vi "运维调试_氨氮.vi"() -> ()   [LabVIEW 2016, in "斯坦道氨氮.lvlib"]
uses:
  <vilib>/Utility/miscctls.llb/LVPointTypeDef.ctl
  <vilib>/Utility/config.llb/NI_LVConfig.lvlib
  <vilib>/ptbypt/NI_PtbyPt.lvlib
panel:
  in  "仪器参数设置":bool
  in  "模块启用":bool
  in  "串口设置":bool
  in  "备用系数一键写入":bool
  in  "公式一键写入":bool
  in  "流程路径":path=path "C:/Users/STD/Documents/斯坦道流程文件/流程.xml"
  in  "曲线模型":cluster{"X^2":dbl, "X":dbl, "B":dbl}(xcontrol)
  out "字符串":string
  in  "质控参数设置":bool
  in  "自动测试量程配置":T1
  out "温度2":sgl
  out "温度1":sgl
  out "ADC":sgl
  out "固件版本号":string
  in  "数组":string[](array[string])
  in  "备用系数写入":bool
  in  "备用系数读取":bool
  in  "备用系数":T2
  in  "量程切换阈值写入":bool
  in  "量程切换阈值读取":bool
  in  "量程切换阈值":cluster{"阈值":dbl, "标液浓度":dbl}
  in  "参数下拉列表":enum16{"总磷", "总氮", "氨氮"}(ring)=enum."氨氮"
  in  "量程下拉列表":enum16{"低量程", "高量程"}(ring)
  in  "测量模式下拉列表":enum16{"水样测量", "零点核查", "跨度核查", "标样核查", "加标回收"}(ring)
  in  "公式":cluster{"X^2":dbl, "X":dbl, "b":dbl}
  in  "写公式":bool
  in  "读公式":bool
  in  "返回":bool
  in  "设置":bool
  out "序列号":string="序列号"
  out "测量数据":T3(xcontrol)
  out "集成报警信息":string
  out "定时启动":bool
  out "运行状态":T4(xcontrol)
  in  "停止":bool
  in  "手动启动":bool
  in  "单步测试":bool
  in  "总磷氨氮调试":u16[](xcontrol)
  out "F3":sgl format="%#.6f"
  out "F2":sgl format="%#.6f"
  out "F1":sgl format="%#.6f"
  out "F0":sgl format="%#.6f"
  out "多列列表框":i32(listbox)
  # "参数设置"
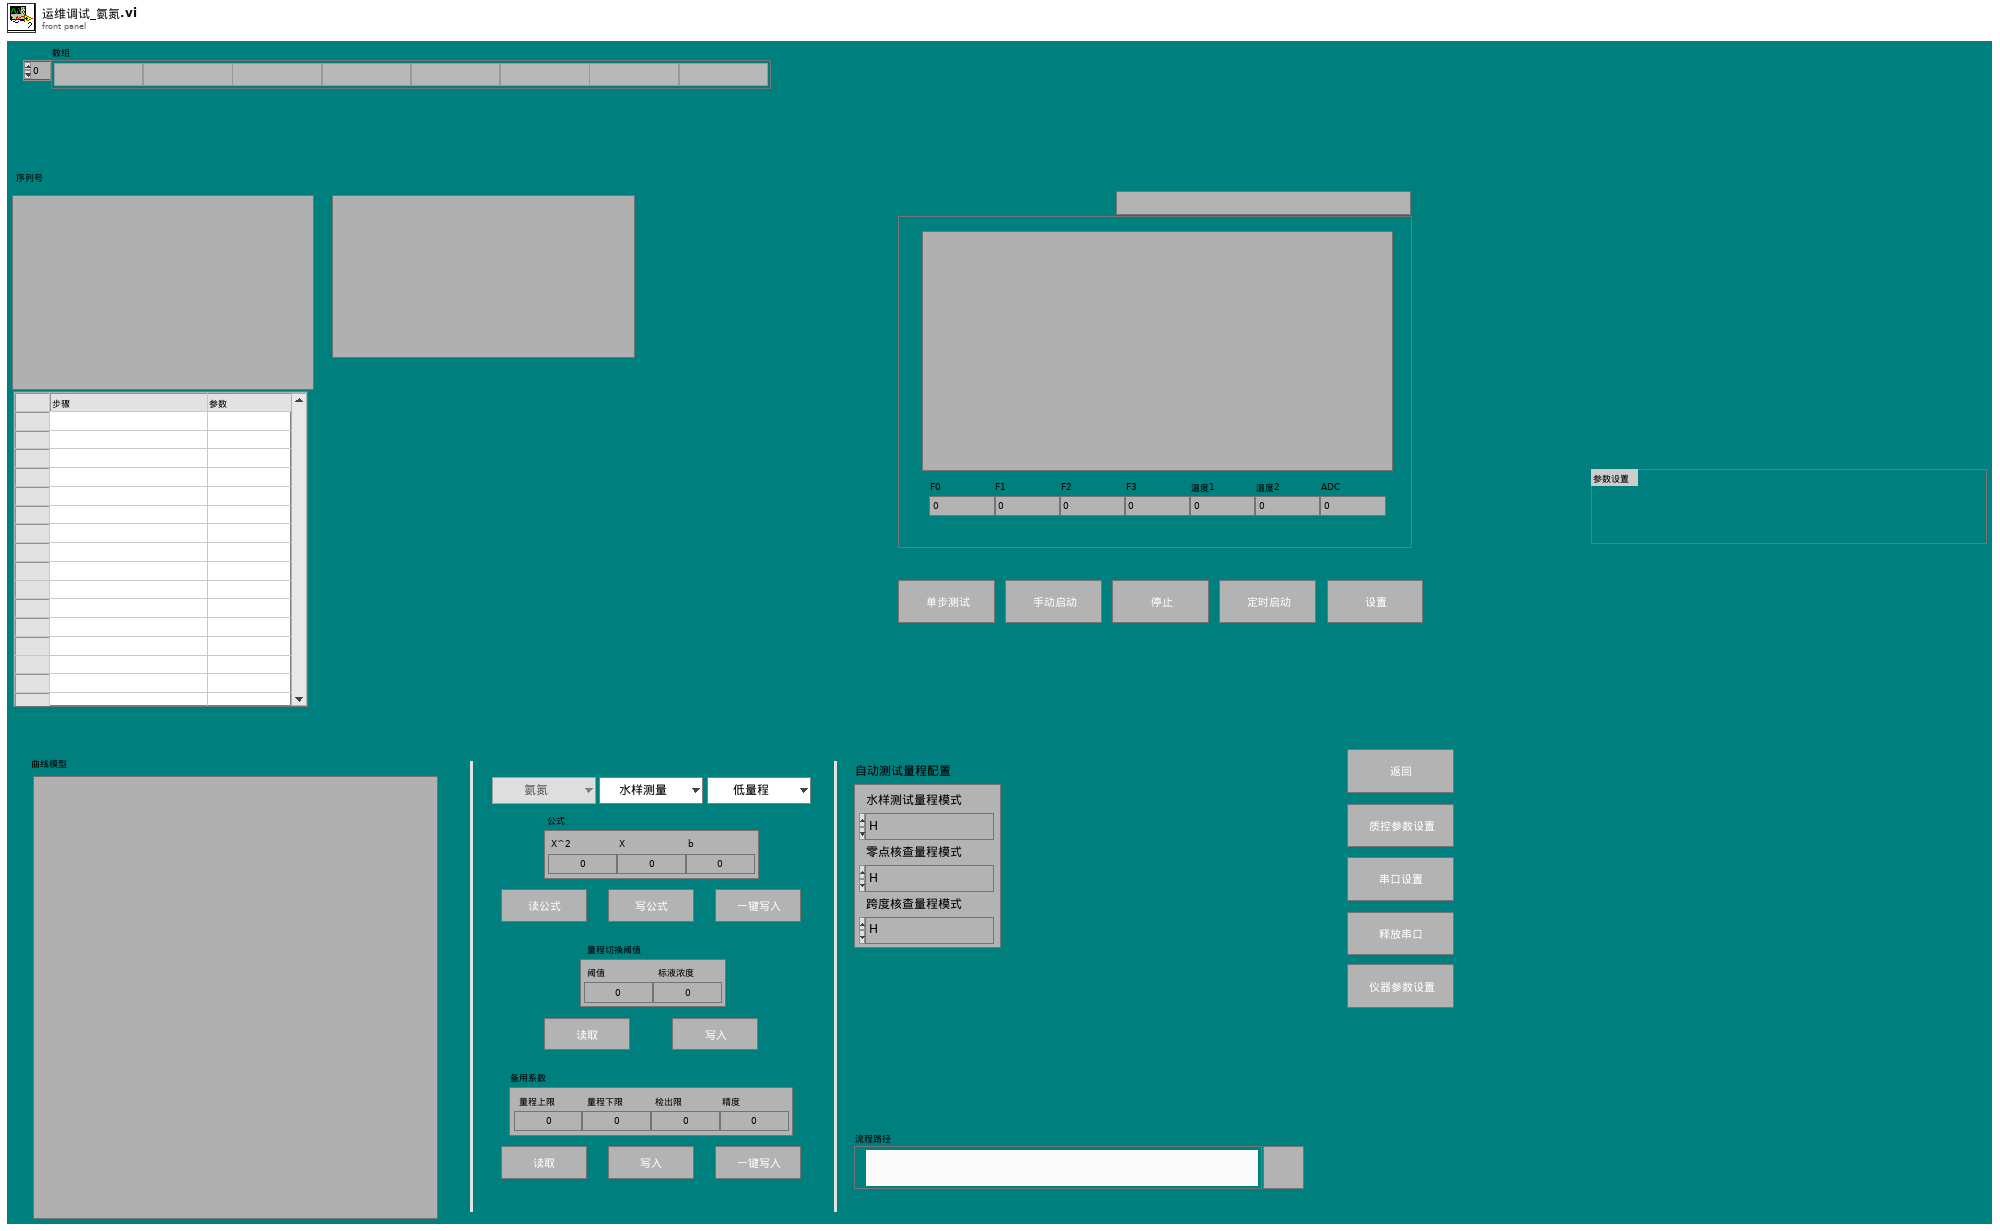
[diagram p1: front panel]
types:
  T1 = cluster{"水样测试量程模式":enum16{"H", "L", "AUTO"}, "空白核查量程模式":enum16{"H", "L", "AUTO"}, "跨度核查量程模式":enum16{"H", "L", "AUTO"}}
  T2 = cluster{"量程上限":dbl, "量程下限":dbl, "检出限":dbl, "精度":dbl}
  T3 = cluster{"flowid":u16, "测量精度":u16, "测量数据区":cluster{"因子编码":u32, "单位":u16, "标样参考值":sgl, "水样数据时间":timestamp, "水样实测值":sgl, "水样数据标识":string, "标样数据时间":timestamp, "标样实测值":sgl, "标样数据标识":string, "空白数据时间":timestamp, "空白实测值":sgl, "空白数据标识":string, "零点核查数据时间":timestamp, "零点核查实测值":sgl, "零点核查数据标识":string, "跨度核查数据时间":timestamp, "跨度核查实测值":sgl, "跨度核查数据标识":string, "加标回收数据时间":timestamp, "加标回收实测值":sgl, "加标回收数据标识":string, "平行样数据时间":timestamp, "平行样实测值":sgl, "平行样数据标识":string, "F0":sgl, "F1":sgl, "F2":sgl, "F3":sgl, "F4":sgl, "F5":sgl, "F6":sgl, "F7":sgl, "温度":sgl, "湿度":sgl, "X值":sgl}}
  T4 = cluster{"系统时间":timestamp, "工作状态":enum16{"空闲", "水样测试", "标样核查", "零点核查", "跨度核查", "空白测试", "平行样测试", "加标回收", "空白校准", "标样校准", "初始化（清洗）"}, "测量模式":enum16{"待机", "连续模式", "周期模式", "定点模式", "受控模式", "手动模式"}, "告警代码":u16, "故障代码":u16, "日志代码":u16, "软件版本":u16, "F0":sgl, "F1":sgl, "F2":sgl, "F3":sgl, "T":sgl, "H":sgl, "id":u16, "flowid":u16, "量程":u16, "总磷控温温度1":sgl, "营养盐控温温度2":sgl, "ADC":sgl}
  T5 = enum16{"启动测量", "标样核查", "零点核查", "跨度核查", "空白测试", "平行样测试", "加标回收", "空白校准", "标样校准", "初始化（清洗）", "停止测试", "仪器重启", "校时", "模式设置", "测量间隔设置"}
  T6 = cluster{"控制命令":enum16{"启动测量", "标样核查", "零点核查", "跨度核查", "空白测试", "平行样测试", "加标回收", "空白校准", "标样校准", "初始化（清洗）", "停止测试", "仪器重启", "校时", "模式设置", "测量间隔设置"}, "周期设置类型":enum16{"定点启动", "间隔启动"}, "定时功能启用":bool, "定时间隔":dbl, "24H周期设置":bool[], "零点核查时间":u16, "跨度核查时间":u16, "质控频次":enum16{"关闭", "每天", "星期一", "星期二", "星期三", "星期四", "星期五", "星期六", "星期日"}}
  T7 = enum16{"关闭", "每天", "星期一", "星期二", "星期三", "星期四", "星期五", "星期六", "星期日"}
  T8 = typedef "LVDateTimeRec.ctl" = cluster{"秒数的小数部分":dbl, "秒":i32, "分":i32, "时":i32, "日":i32, "月":i32, "年":i32, "天数（周）":i32, "天数（年）":i32, "DST":i32}
  T9 = enum16{"空闲", "水样测试", "标样核查", "零点核查", "跨度核查", "空白测试", "平行样测试", "加标回收", "空白校准", "标样校准", "初始化（清洗）"}
  T10 = enum32{"Bad", "Idle", "Run top level", "Running"}
  T11 = typedef "LVPointTypeDef.ctl" = cluster{"Horizontal":i16, "Vertical":i16}
  T12 = cluster{"因子编码":u32, "单位":u16, "标样参考值":sgl, "水样数据时间":timestamp, "水样实测值":sgl, "水样数据标识":string, "标样数据时间":timestamp, "标样实测值":sgl, "标样数据标识":string, "空白数据时间":timestamp, "空白实测值":sgl, "空白数据标识":string, "零点核查数据时间":timestamp, "零点核查实测值":sgl, "零点核查数据标识":string, "跨度核查数据时间":timestamp, "跨度核查实测值":sgl, "跨度核查数据标识":string, "加标回收数据时间":timestamp, "加标回收实测值":sgl, "加标回收数据标识":string, "平行样数据时间":timestamp, "平行样实测值":sgl, "平行样数据标识":string, "F0":sgl, "F1":sgl, "F2":sgl, "F3":sgl, "F4":sgl, "F5":sgl, "F6":sgl, "F7":sgl, "温度":sgl, "湿度":sgl, "X值":sgl}
  T13 = typedef "NI_LVConfig.lvlib/Config Data RefNum.ctl" = refnum<k1>
  T14 = cluster{"参数下拉列表":enum16{"总磷", "总氮", "氨氮"}, "测量模式下拉列表":enum16{"水样测量", "零点核查", "跨度核查", "标样核查", "加标回收"}, "量程下拉列表":enum16{"低量程", "高量程"}}
  T15 = cluster{"启动模式":enum16{"跨度核查", "水样测量", "空白核查", "标样核查", "加标回收"}, "启动参数":u16, "量程":enum16{"低量程", "高量程"}}
  T16 = cluster{"时间标识":timestamp, "设备":string, "日志信息":string, "流程参数":string}
  T17 = cluster{"时间标识":timestamp, "设备":string, "日志信息":string}
  T18 = typedef "LVRowAndColumnUnsignedTypeDef.ctl" = cluster{"Row":u32, "Column":u32}
  T19 = cluster{"站号":u16, "量程切换":enum32{"H", "L", "AUTO"}, "控制命令":enum16{"启动测量", "标样核查", "零点核查", "跨度核查", "空白测试", "平行样测试", "加标回收", "空白校准", "标样校准", "初始化（清洗）", "停止测试", "仪器重启", "校时", "模式设置", "测量间隔设置"}, "模式设置":enum16{"待机", "连续模式", "周期模式", "定点模式", "受控模式", "手动模式"}, "测量间隔":u16}
  T20 = cluster{"氨氮跨度值":dbl, "氨氮零点标准液浓度":dbl, "氨氮跨度标准液浓度":dbl, "氨氮标准液标准浓度":dbl}
  T21 = cluster{"确定":bool, "跨度值":dbl, "零点标准液浓度":dbl, "跨度标准液浓度":dbl, "标准液标准浓度":dbl}
  T22 = cluster{"测量量程":dbl, "测量精度":dbl, "测量间隔":dbl, "消解温度":dbl, "消解时长":dbl, "空白校准时间":timestamp, "曲线截距":dbl, "曲线斜率":dbl, "测量检出限":dbl, "测量信号值":dbl, "线性相关系数":dbl, "二次多项式系数":dbl, "标样校准时间":timestamp, "单位":u16}
  T23 = cluster{"确定":bool, "测量量程":dbl, "测量精度":dbl, "测量间隔":dbl, "消解温度":dbl, "消解时长":dbl, "空白校准时间":timestamp, "曲线截距":dbl, "曲线斜率":dbl, "测量检出限":dbl, "测量信号值":dbl, "线性相关系数":dbl, "二次多项式系数":dbl, "标样校准时间":timestamp, "单位":u16}
  T24 = cluster{"控制命令":enum16{"启动测量", "标样核查", "零点核查", "跨度核查", "空白测试", "平行样测试", "加标回收", "空白校准", "标样校准", "初始化（清洗）", "停止测试", "仪器重启", "校时", "模式设置", "测量间隔设置"}, "周期设置类型":enum16{"定点启动", "间隔启动"}, "定时功能启用":bool, "定时间隔":dbl, "24H周期设置":bool[], "空白核查时间":u16, "跨度核查时间":u16, "质控频次":enum16{"关闭", "每天", "星期一", "星期二", "星期三", "星期四", "星期五", "星期六", "星期日"}}
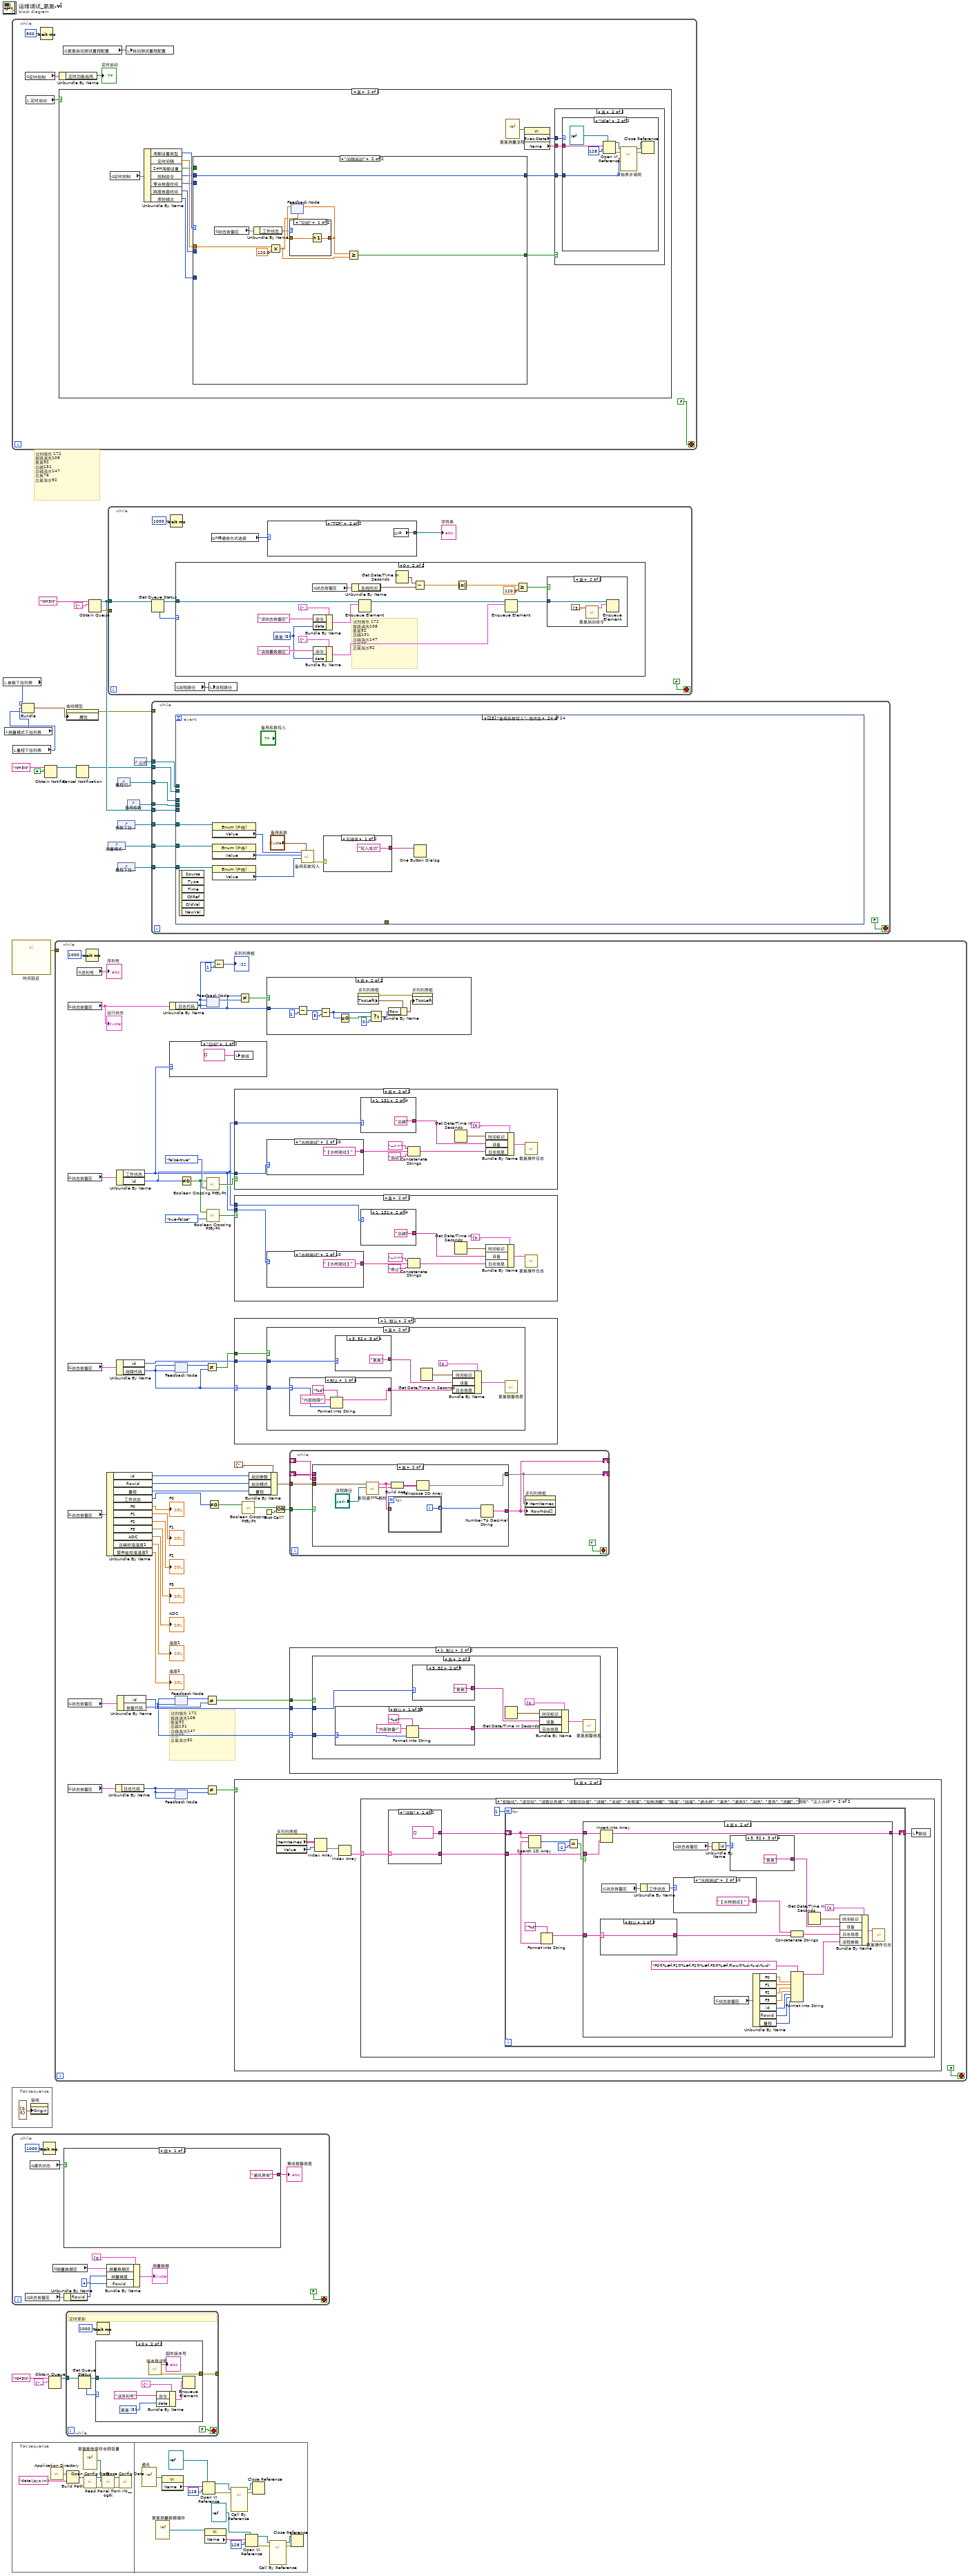
[diagram p0: block diagram]
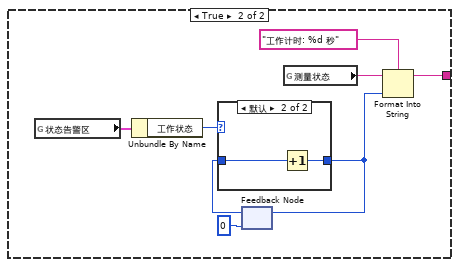
[diagram p3: hidden frame]
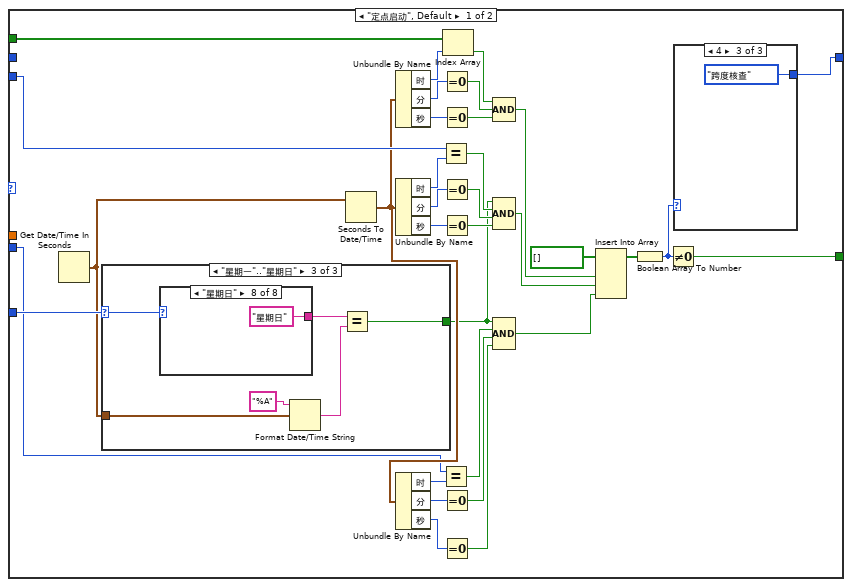
[diagram p8: hidden frame]
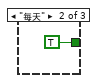
[diagram p10: hidden frame]
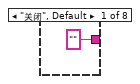
[diagram p11: hidden frame]
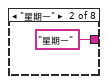
[diagram p12: hidden frame]
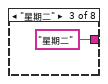
[diagram p13: hidden frame]
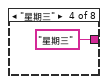
[diagram p14: hidden frame]
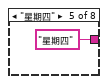
[diagram p15: hidden frame]
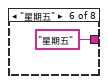
[diagram p16: hidden frame]
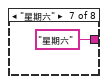
[diagram p17: hidden frame]
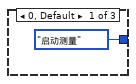
[diagram p18: hidden frame]
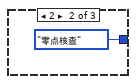
[diagram p19: hidden frame]
diagram:
  # "试剂填充 172 \n管路清洗108\n氨氮92\n总磷131\n总磷海水147\n总氮76\n总氮海水92"
  n1 = local read "参数下拉列表"() -> (w4:enum16{"总磷", "总氮", "氨氮"})
  n2 = local read "测量模式下拉列表"() -> (w3:enum16{"水样测量", "零点核查", "跨度核查", "标样核查", "加标回收"})
  n3 = while {
    stop <- FALSE stop-if-true
    n4 = global read "氨氮断电保存全局变量.vi" "定时控制"() -> (w25:T6)
    n5 = local read "定时启动"() -> (w27:bool)
    n6 = Wait (ms)(milliseconds to wait=u32 500 ("等待时间（毫秒）")) -> ()  [unwired: 1 out]
    n7 = Unbundle By Name(w25) -> ("定时功能启用"=→"定时启动":bool)
    n8 = case shown="真" w27 {
      frame False {
      }
      frame True {
        n9 = global read "氨氮断电保存全局变量.vi" "定时控制"() -> (w42:T6)
        n10 = Unbundle By Name(w42) -> ("周期设置类型"=w41:enum16{"定点启动", "间隔启动"}, "定时间隔"=w40:dbl, "24H周期设置"=w39:bool[], "控制命令"=w34:T5, "零点核查时间"=w32:u16, "跨度核查时间"=w31:u16, "质控频次"=w30:T7)
        n11 = case shown="\"间隔启动\"" w41 {
          tunnel: w40 -> [_ w111]
          tunnel: w39 -> [w77 _]
          tunnel: [w55 w109] -> w38
          tunnel: w34 -> [_ w107]
          tunnel: [w81 w107] -> w33
          tunnel: w30 -> [w80 _]
          tunnel: w32 -> [w73 _]
          tunnel: w31 -> [w62 _]
          frame "定点启动", Default {
            n12 = Get Date/Time In Seconds() -> (seconds since 1Jan1904=w79:timestamp)
            n13 = case shown="\"星期一\"..\"星期日\"" w80 {
              selector: w80 -> [_ _ w91]
              tunnel: w79 -> [_ _ w92]
              tunnel: [_ TRUE w88] -> w61
              frame "关闭", Default {
              }
              frame "每天" {
              }
              frame "星期一".."星期日" {
                n14 = case shown="\"星期日\"" w91 {
                  tunnel: ["" ("时间格式字符串(%c)") "星期一" ("时间格式字符串(%c)") "星期二" ("时间格式字符串(%c)") "星期三" ("时间格式字符串(%c)") "星期四" ("时间格式字符串(%c)") "星期五" ("时间格式字符串(%c)") "星期六" ("时间格式字符串(%c)") "星期日" ("时间格式字符串(%c)")] -> w90
                  frame "关闭", Default {
                  }
                  frame "星期一" {
                  }
                  frame "星期二" {
                  }
                  frame "星期三" {
                  }
                  frame "星期四" {
                  }
                  frame "星期五" {
                  }
                  frame "星期六" {
                  }
                  frame "星期日" {
                  }
                }
                n15 = Format Date/Time String(time format string (%c)="%A" ("时间格式字符串(%c)"), seconds (now)=w92) -> (date/time string=w89:string)  [unwired: 1 in]
                n16 = Equal?(x=w90, y=w89) -> (x = y?=w88:bool)
              }
            }
            n17 = Seconds To Date/Time(time stamp (now)=w79) -> (date time rec=w63:T8)  [unwired: 1 in]
            n18 = Unbundle By Name(w63) -> ("时"=w86:i32, "分"=w84:i32, "秒"=w85:i32)
            n19 = Unbundle By Name(w63) -> ("时"=w74:i32, "分"=w76:i32, "秒"=w75:i32)
            n20 = Unbundle By Name(w63) -> ("时"=w66:i32, "分"=w64:i32, "秒"=w65:i32)
            n21 = Equal?(x=w73, y=w74) -> (x = y?=w72:bool)
            n22 = Equal?(x=w62, y=w66) -> (x = y?=w67:bool)
            n23 = Equal To 0?(x=w84) -> (x = 0?=w83:bool)
            n24 = Equal To 0?(x=w85) -> (x = 0?=w82:bool)
            n25 = Equal To 0?(x=w76) -> (x = 0?=w71:bool)
            n26 = Equal To 0?(x=w75) -> (x = 0?=w70:bool)
            n27 = Equal To 0?(x=w64) -> (x = 0?=w68:bool)
            n28 = Equal To 0?(x=w65) -> (x = 0?=w69:bool)
            n29 = Index Array(array=w77, index=w86) -> (element=w78:bool)
            n30 = Compound Arithmetic op=AND ("复合运算")(w78, w83, w82) -> (w59:bool)
            n31 = Compound Arithmetic op=AND ("复合运算")(w61, w72, w71, w70) -> (w58:bool)
            n32 = Compound Arithmetic op=AND ("复合运算")(w61, w67, w68, w69) -> (w57:bool)
            n33 = Insert Into Array(array=bool[] [], new element #1=w59, new element #2=w58, new element #3=w57) -> (w56:bool[])  [unwired: 1 in]
            n34 = Boolean Array To Number(Boolean array=w56) -> (number=w54:u32)
            n35 = Not Equal To 0?(x=w54) -> (x != 0?=w55:bool)
            n36 = case shown="4" w54 {
              tunnel: [T5."启动测量" ("控制命令") T5."零点核查" ("控制命令") T5."跨度核查" ("控制命令")] -> w81
              frame 0, Default {
              }
              frame 2 {
              }
              frame 4 {
              }
            }
          }
          frame "间隔启动" {
            n37 = global read "VAR氨氮全局变量.vi" "状态告警区"() -> (w106:T4)
            n38 = Unbundle By Name(w106) -> ("工作状态"=w105:T9)
            n39 = Multiply(x=w111, y=120.0) -> (x*y=w108:dbl)
            n40 = feedback #1(w108) -> (w113:dbl)
            n41 = case shown="\"空闲\"" w105 {
              tunnel: w113 -> [w115 _]
              tunnel: [w114 _] -> w112
              frame "空闲" {
                n42 = Increment(x=w115) -> (x+1=w114:dbl)
              }
              frame "水样测试", Default {
              }
            }
            n43 = feedback-in #1(w112) -> ()
            n44 = Greater Or Equal?(x=w112, y=w108) -> (x >= y?=w109:bool)
          }
        }
        n45 = vi-ref "氨氮测量流程.vi"() -> (w37:refnum<vi>)
        n46 = property class="VI"(reference=w37) -> ("Exec.State"=w36:T10, "Name"=w35:string)  [unwired: 1 in, 2 out]
        n47 = case shown="真" w38 {
          tunnel: w35 -> [_ w45]
          tunnel: w33 -> [_ w44]
          tunnel: w36 -> [_ w43]
          frame False {
          }
          frame True {
            n48 = case shown="\"Idle\"" w43 {
              tunnel: w45 -> [_ w49]
              tunnel: w44 -> [_ w47]
              frame "Bad", Default {
              }
              frame "Idle" {
                n49 = Open VI Reference(type specifier VI Refnum (for type only)=refnum<vi> refnum, vi path=w49, options=128 ("选项")) -> (vi reference=w50:refnum<vi>, error out=w51:errorcluster)  [unwired: 3 in]
                n50 = call-by-ref "开始异步调用"(reference=w50, error in=w51, "控制命令"=w47) -> (reference out=w52:refnum<vi>, error out=w53:errorcluster)  [unwired: 11 in]
                n51 = Close Reference(reference=w52, error in (no error)=w53) -> ()  [unwired: 1 out]
              }
            }
          }
        }
      }
    }
    n52 = global read "氨氮断电保存全局变量.vi" "氨氮自动测试量程配置"() -> (w26:T1)
    n53 = local write "自动测试量程配置"(w26) -> ()
  }
  n54 = call "时间延迟"() -> ("error out"=w13:errorcluster)  [unwired: 11 in]
  n55 = flat-sequence {
    frame #0 {
      n56 = property on="窗格" class="Pane"("Origin"=T11 {"Horizontal"=0, "Vertical"=0} ("原点")) -> ()  [unwired: 2 in, 2 out]
    }
  }
  n57 = while {
    stop <- FALSE stop-if-true
    n58 = global read "VAR氨氮全局变量.vi" "状态告警区"() -> (w122:T4)
    n59 = global read "VAR氨氮全局变量.vi" "通讯状态"() -> (w124:bool)
    n60 = Wait (ms)(milliseconds to wait=u32 1000 ("等待时间（毫秒）")) -> ()  [unwired: 1 out]
    n61 = global read "VAR氨氮全局变量.vi" "测量数据区"() -> (w117:T12)
    n62 = case shown="假" w124 {
      tunnel: ["通讯异常" ("集成报警信息") w129] -> w123
      frame False {
      }
      frame True {
        n63 = global read "VAR氨氮全局变量.vi" "状态告警区"() -> (w135:T4)
        n64 = Unbundle By Name(w135) -> ("工作状态"=w134:T9)
        n65 = feedback #2(0) -> (w132:i32)
        n66 = case shown="默认" w134 {
          tunnel: w132 -> [_ w137]
          tunnel: [_ w136] -> w130
          frame "空闲" {
          }
          frame Default {
            n67 = Increment(x=w137) -> (x+1=w136:i32)
          }
        }
        n68 = feedback-in #2(w130) -> ()
        n69 = global read "VAR氨氮全局变量.vi" "测量状态"() -> (w128:string)
        n70 = Format Into String(format string="工作计时: %d 秒" ("格式字符串"), initial string=w128, w130) -> (resulting string=w129:string)  [unwired: 1 in, 1 out]
      }
    }
    "集成报警信息" <- w123
    n71 = Unbundle By Name(w122) -> ("flowid"=w121:u16)
    n72 = Bundle By Name(cluster=T3 {"flowid"=0, "测量精度"=0, "测量数据区"={"因子编码"=0, "单位"=0, "标样参考值"=0.0, "水样数据时间"=timestamp(0 s since 1904-01-01), "水样实测值"=0.0, "水样数据标识"="", "标样数据时间"=timestamp(0 s since 1904-01-01), "标样实测值"=0.0, "标样数据标识"="", "空白数据时间"=timestamp(0 s since 1904-01-01), "空白实测值"=0.0, "空白数据标识"="", "零点核查数据时间"=timestamp(0 s since 1904-01-01), "零点核查实测值"=0.0, "零点核查数据标识"="", "跨度核查数据时间"=timestamp(0 s since 1904-01-01), "跨度核查实测值"=0.0, "跨度核查数据标识"="", "加标回收数据时间"=timestamp(0 s since 1904-01-01), "加标回收实测值"=0.0, "加标回收数据标识"="", "平行样数据时间"=timestamp(0 s since 1904-01-01), "平行样实测值"=0.0, "平行样数据标识"="", "F0"=0.0, "F1"=0.0, "F2"=0.0, "F3"=0.0, "F4"=0.0, "F5"=0.0, "F6"=0.0, "F7"=0.0, "温度"=0.0, "湿度"=0.0, "X值"=0.0}} ("总氮测量数据"), "测量数据区"=w117, "测量精度"=u16 4, "flowid"=w121) -> (→"测量数据":T3)
  }
  n73 = flat-sequence {
    frame #0 {
      n74 = call <vilib>:"Application Directory.vi"() -> ("Application Directory"=w145:path)
      n75 = Build Path(base path=w145, name or relative path="data\\sys.ini" ("名称或相对路径")) -> (appended path=w143:path)
      n76 = vi-ref "氨氮断电保存全局变量.vi"() -> (w141:refnum<vi>)
      n77 = call <vilib>:"Open Config Data.vi"("configuration file path"=w143) -> ("error out"=w139:errorcluster, "refnum"=w142:T13)  [unwired: 8 in, 1 out]
      n78 = call <userlib>:"Read Panel from INI__ogtk.vi"("error in (no error)"=w139, "VI ref"=w141, "refnum"=w142) -> ("error out"=w138:errorcluster, "refnum out"=w140:T13)  [unwired: 7 in]
      n79 = call <vilib>:"Close Config Data.vi"("error in (no error)"=w138, "refnum"=w140) -> ()  [unwired: 8 in, 2 out]
    }
    frame #1 {
      n80 = vi-ref "通讯.vi"() -> (w161:refnum<vi>)
      n81 = vi-ref "氨氮测量数据储存.vi"() -> (w153:refnum<vi>)
      n82 = property class="VI"(reference=w161) -> ("Name"=w160:string)  [unwired: 1 in, 2 out]
      n83 = Open VI Reference(type specifier VI Refnum (for type only)=refnum<vi> refnum, vi path=w160, options=128 ("选项")) -> (vi reference=w158:refnum<vi>, error out=w156:errorcluster)  [unwired: 3 in]
      n84 = property class="VI"(reference=w153) -> ("Name"=w146:string)  [unwired: 1 in, 2 out]
      n85 = call-by-ref "?"(reference=w158, error in=w156) -> (reference out=w154:refnum<vi>, error out=w155:errorcluster)  [unwired: 12 in]
      n86 = Open VI Reference(type specifier VI Refnum (for type only)=refnum<vi> refnum, vi path=w146, options=128 ("选项")) -> (vi reference=w148:refnum<vi>, error out=w150:errorcluster)  [unwired: 3 in]
      n87 = Close Reference(reference=w154, error in (no error)=w155) -> ()  [unwired: 1 out]
      n88 = call-by-ref "?"(reference=w148, error in=w150) -> (reference out=w152:refnum<vi>, error out=w151:errorcluster)  [unwired: 12 in]
      n89 = Close Reference(reference=w152, error in (no error)=w151) -> ()  [unwired: 1 out]
    }
  }
  n90 = local read "量程下拉列表"() -> (w2:enum16{"低量程", "高量程"})
  n91 = Bundle("参数下拉列表"=w4, "测量模式下拉列表"=w3, "量程下拉列表"=w2) -> (w1:T14)  [unwired: 1 in]
  n92 = Obtain Notifier(name (unnamed)="NH3N" ("名称（未命名）"), notification data type=FALSE) -> (notifier out=w6:refnum<notifier>)  [unwired: 2 in, 2 out]
  n93 = Obtain Queue(name (unnamed)="NH3N" ("名称（未命名）"), element data type=cluster{"命令":string, "data":variant} {"命令"="", "data"=variant}) -> (queue out=w10:refnum<queue>)  [unwired: 3 in, 2 out]
  n94 = while {
    tunnel: w13 -> [_]
    stop <- FALSE stop-if-true
    # "试剂填充 172 \n管路清洗108\n氨氮92\n总磷131\n总磷海水147\n总氮76\n总氮海水92"
    n95 = global read "VAR氨氮全局变量.vi" "状态告警区"() -> (w195:T4)
    "运行状态" <- w195
    n96 = global read "VAR氨氮全局变量.vi" "状态告警区"() -> (w182:T4)
    n97 = global read "VAR氨氮全局变量.vi" "状态告警区"() -> (w187:T4)
    n98 = global read "VAR氨氮全局变量.vi" "状态告警区"() -> (w203:T4)
    n99 = global read "VAR氨氮全局变量.vi" "状态告警区"() -> (w192:T4)
    n100 = global read "VAR氨氮全局变量.vi" "状态告警区"() -> (w180:T4)
    n101 = global read "VAR氨氮全局变量.vi" "序列号"() -> (→"序列号":string)
    n102 = Wait (ms)(milliseconds to wait=u32 1000 ("等待时间（毫秒）")) -> ()  [unwired: 1 out]
    n103 = Unbundle By Name(w203) -> ("id"=w200:u16, "flowid"=w202:u16, "量程"=w201:u16, "工作状态"=w170:T9, "F0"=→"F0":sgl, "F1"=→"F1":sgl, "F2"=→"F2":sgl, "F3"=→"F3":sgl, "ADC"=→"ADC":sgl, "总磷控温温度1"=→"温度1":sgl, "营养盐控温温度2"=→"温度2":sgl)
    n104 = Unbundle By Name(w180) -> ("日志代码"=w179:u16)
    n105 = Unbundle By Name(w182) -> ("工作状态"=w166:T9, "id"=w165:u16)
    n106 = Unbundle By Name(w187) -> ("id"=w186:u16, "故障代码"=w183:u16)
    n107 = Unbundle By Name(w192) -> ("id"=w191:u16, "告警代码"=w188:u16)
    n108 = Unbundle By Name(w195) -> ("日志代码"=w176:u16)
    n109 = case shown="\"空闲\"" w166 {
      frame "空闲" {
        n110 = local write "数组"(string[] [] ("数组")) -> ()
      }
      frame "水样测试", Default {
      }
    }
    n111 = feedback #3(w183) -> (w184:u16)
    n112 = feedback-in #3(w183) -> ()
    n113 = feedback #4(w188) -> (w189:u16)
    n114 = feedback-in #4(w188) -> ()
    n115 = feedback #5(w179) -> (w181:u16)
    n116 = feedback-in #5(w179) -> ()
    n117 = Not Equal To 0?(x=w165) -> (x != 0?=w163:bool)
    n118 = Not Equal?(x=w184, y=w183) -> (x != y?=w185:bool)
    n119 = Not Equal?(x=w189, y=w188) -> (x != y?=w190:bool)
    n120 = Not Equal?(x=w179, y=w181) -> (x != y?=w178:bool)
    n121 = feedback-in #6(w176) -> ()
    n122 = feedback #6(w176) -> (w208:u16)
    n123 = call <vilib>:"Boolean Crossing PtByPt.vi"("direction"=enum16{"either", "false-true", "true-false"}."false-true", "input"=w163) -> ("crossing"=w167:bool)  [unwired: 1 in]
    n124 = call <vilib>:"Boolean Crossing PtByPt.vi"("direction"=enum16{"either", "false-true", "true-false"}."true-false", "input"=w163) -> ("crossing"=w162:bool)  [unwired: 1 in]
    n125 = Not Equal To 0?(x=w170) -> (x != 0?=w205:bool)
    n126 = Subtract(x=w176, y=1) -> (x-y=→"多列列表框":i32)
    n127 = case shown="真" w167 {
      tunnel: w165 -> [_ w235]
      tunnel: w166 -> [_ w234]
      frame False {
      }
      frame True {
        n128 = case shown="\"水样测试\"" w234 {
          tunnel: [_ "【水样测试】" ("字符串") "【标样核查】" ("字符串") "【零点核查】" ("字符串") "【跨度核查】" ("字符串") "【空白测试】" ("字符串") "【平行样测试】" ("字符串") "【加标回收】" ("字符串") "【空白校准】" ("字符串") "【标样校准】" ("字符串")] -> w239
          frame "空闲", Default {
          }
          frame "水样测试" {
          }
          frame "标样核查" {
          }
          frame "零点核查" {
          }
          frame "跨度核查" {
          }
          frame "空白测试" {
          }
          frame "平行样测试" {
          }
          frame "加标回收" {
          }
          frame "空白校准" {
          }
          frame "标样校准" {
          }
        }
        n129 = case shown="1, 131" w235 {
          tunnel: [_ "总磷" ("table输入") "氨氮" ("table输入") "总氮" ("table输入")] -> w240
          frame Default {
          }
          frame 1, 131 {
          }
          frame 3, 92 {
          }
          frame 2, 76 {
          }
        }
        n130 = Concatenate Strings("-->>" ("字符串"), w239, "启动" ("字符串")) -> (w238:string)
        n131 = Get Date/Time In Seconds() -> (seconds since 1Jan1904=w241:timestamp)
        n132 = Bundle By Name(cluster=T16 {"时间标识"=timestamp(0 s since 1904-01-01), "设备"="", "日志信息"="", "流程参数"=""} ("data in"), "时间标识"=w241, "设备"=w240, "日志信息"=w238) -> (w233:T16)
        n133 = call "氨氮操作日志.vi"("data in"=w233) -> ()  [unwired: 11 in]
      }
    }
    n134 = case shown="真" w162 {
      tunnel: w165 -> [_ w213]
      tunnel: w166 -> [_ w212]
      frame False {
      }
      frame True {
        n135 = case shown="\"水样测试\"" w212 {
          tunnel: [_ "【水样测试】" ("字符串") "【标样核查】" ("字符串") "【零点核查】" ("字符串") "【跨度核查】" ("字符串") "【空白测试】" ("字符串") "【平行样测试】" ("字符串") "【加标回收】" ("字符串") "【空白校准】" ("字符串") "【标样校准】" ("字符串")] -> w217
          frame "空闲", Default {
          }
          frame "水样测试" {
          }
          frame "标样核查" {
          }
          frame "零点核查" {
          }
          frame "跨度核查" {
          }
          frame "空白测试" {
          }
          frame "平行样测试" {
          }
          frame "加标回收" {
          }
          frame "空白校准" {
          }
          frame "标样校准" {
          }
        }
        n136 = case shown="1, 131" w213 {
          tunnel: [_ "总磷" ("table输入") "氨氮" ("table输入") "总氮" ("table输入")] -> w218
          frame Default {
          }
          frame 1, 131 {
          }
          frame 3, 92 {
          }
          frame 2, 76 {
          }
        }
        n137 = Concatenate Strings("-->>" ("字符串"), w217, "停止" ("字符串")) -> (w216:string)
        n138 = Get Date/Time In Seconds() -> (seconds since 1Jan1904=w219:timestamp)
        n139 = Bundle By Name(cluster=T16 {"时间标识"=timestamp(0 s since 1904-01-01), "设备"="", "日志信息"="", "流程参数"=""} ("data in"), "时间标识"=w219, "设备"=w218, "日志信息"=w216) -> (w211:T16)
        n140 = call "氨氮操作日志.vi"("data in"=w211) -> ()  [unwired: 11 in]
      }
    }
    n141 = case shown="1, 默认" w183 {
      selector: w183 -> [_ w323]
      tunnel: w186 -> [_ w324]
      tunnel: w185 -> [_ w322]
      frame 0 {
      }
      frame 1, Default {
        n142 = case shown="真" w322 {
          tunnel: w324 -> [_ w331]
          tunnel: w323 -> [_ w326]
          frame False {
          }
          frame True {
            n143 = case shown="默认" w326 {
              selector: w326 -> [w333 _ _ _ _ _]
              tunnel: [w332 "无故障" "电机故障" "温度故障" "通讯故障" "滴定故障"] -> w325
              frame Default {
                n144 = Format Into String(format string="%d" ("格式字符串"), initial string="内部故障-" ("工作状态"), w333) -> (resulting string=w332:string)  [unwired: 1 in, 1 out]
              }
              frame 0 {
              }
              frame 1 {
              }
              frame 2 {
              }
              frame 3 {
              }
              frame 4 {
              }
            }
            n145 = case shown="3, 92" w331 {
              tunnel: [_ "总磷" ("table输入") "氨氮" ("table输入") "总氮" ("table输入")] -> w327
              frame Default {
              }
              frame 1, 131 {
              }
              frame 3, 92 {
              }
              frame 2, 76 {
              }
            }
            n146 = Get Date/Time In Seconds() -> (seconds since 1Jan1904=w328:timestamp)
            n147 = Bundle By Name(cluster=T17 {"时间标识"=timestamp(0 s since 1904-01-01), "设备"="", "日志信息"=""} ("data in"), "时间标识"=w328, "设备"=w327, "日志信息"=w325) -> (w329:T17)
            n148 = call "氨氮报警信息.vi"("data in"=w329) -> ()  [unwired: 10 in, 1 out]
          }
        }
      }
    }
    n149 = case shown="真" w178 {
      frame False {
      }
      frame True {
        n150 = property on="多列列表框" class="MCListbox (严格)"() -> ("ItemNames"=w258:string[][], "Value"=w259:i32)  [unwired: 2 in, 2 out]
        n151 = Index Array(array=w258, index (row)=w259) -> (element=w257:string[])  [unwired: 1 in]
        n152 = Index Array(array=w257) -> (element=w256:string)  [unwired: 1 in]
        n153 = case shown="\"初始化\", \"读空白\", \"读取比色值\", \"读取空白值\", \"读数\", \"关阀\", \"关恒温\", \"加热消解\", \"降温\", \"结束\", \"进水样\", \"清洗\", \"清洗1\", \"润洗\", \"显色\", \"消解\", \"预热\", \"注入水样\"" w256 {
          selector: w256 -> [_ w262]
          frame Default {
          }
          frame "初始化", "读空白", "读取比色值", "读取空白值", "读数", "关阀", "关恒温", "加热消解", "降温", "结束", "进水样", "清洗", "清洗1", "润洗", "显色", "消解", "预热", "注入水样" {
            n154 = case shown="\"读数\"" w262 {
              selector: w262 -> [w266 w268]
              tunnel: [w266 w268] -> w261
              tunnel: [string[] [] ("数组") "数组"] -> w260
              frame "读数" {
              }
              frame Default {
              }
            }
            n155 = for {
              N: 1 -> [_]
              tunnel: w261 -> [w270]
              shift-right: [w269] -> w263
              shift-left: w260 -> [w271]
              n156 = Search 1D Array(1D array=w271, element=w270) -> (index of element=w274:i32)  [unwired: 1 in]
              n157 = Format Into String(format string="%s" ("格式字符串"), w270) -> (resulting string=w275:string)  [unwired: 2 in, 1 out]
              n158 = Equal?(x=w274, y=-1) -> (x = y?=w272:bool)
              n159 = case shown="真" w272 {
                tunnel: w275 -> [_ w283]
                tunnel: w271 -> [w277 w287]
                tunnel: w270 -> [_ w286]
                tunnel: [w277 w285] -> w269
                frame False {
                }
                frame True {
                  n160 = Insert Into Array(array=w287, new element=w286) -> (w285:string[])  [unwired: 1 in]
                  n161 = case shown="默认" w283 {
                    selector: w283 -> [w312 w315 w318]
                    tunnel: [w312 w314 w317] -> w282
                    frame Default {
                    }
                    frame "初始化" {
                      n162 = Concatenate Strings("-->>" ("字符串"), w315) -> (w314:string)
                    }
                    frame "结束" {
                      n163 = Concatenate Strings("-->>" ("字符串"), w318) -> (w317:string)
                    }
                  }
                  n164 = global read "VAR氨氮全局变量.vi" "状态告警区"() -> (w281:T4)
                  n165 = Unbundle By Name(w281) -> ("工作状态"=w280:T9)
                  n166 = global read "VAR氨氮全局变量.vi" "状态告警区"() -> (w302:T4)
                  n167 = case shown="\"水样测试\"" w280 {
                    tunnel: [_ "【水样测试】" ("字符串") "【标样核查】" ("字符串") "【零点核查】" ("字符串") "【跨度核查】" ("字符串") "【空白测试】" ("字符串") "【平行样测试】" ("字符串") "【加标回收】" ("字符串") "【空白校准】" ("字符串") "【标样校准】" ("字符串")] -> w278
                    frame "空闲", Default {
                    }
                    frame "水样测试" {
                    }
                    frame "标样核查" {
                    }
                    frame "零点核查" {
                    }
                    frame "跨度核查" {
                    }
                    frame "空白测试" {
                    }
                    frame "平行样测试" {
                    }
                    frame "加标回收" {
                    }
                    frame "空白校准" {
                    }
                    frame "标样校准" {
                    }
                  }
                  n168 = Unbundle By Name(w302) -> ("id"=w301:u16)
                  n169 = global read "VAR氨氮全局变量.vi" "状态告警区"() -> (w297:T4)
                  n170 = case shown="3, 92" w301 {
                    tunnel: [_ "总磷" ("table输入") "氨氮" ("table输入") "总氮" ("table输入")] -> w299
                    frame Default {
                    }
                    frame 1, 131 {
                    }
                    frame 3, 92 {
                    }
                    frame 2, 76 {
                    }
                  }
                  n171 = Unbundle By Name(w297) -> ("F0"=w294:sgl, "F1"=w293:sgl, "F2"=w292:sgl, "F3"=w291:sgl, "id"=w290:u16, "flowid"=w289:u16, "量程"=w288:u16)
                  n172 = Concatenate Strings(w278, w282) -> (w279:string)
                  n173 = Format Into String(format string="F0=%#f,F1=%#f,F2=%#f,F3=%#f,Flow=%d-%-d-%-d" ("格式字符串"), w294, w293, w292, w291, w290, w289, w288) -> (resulting string=w295:string)  [unwired: 2 in, 1 out]
                  n174 = Get Date/Time In Seconds() -> (seconds since 1Jan1904=w298:timestamp)
                  n175 = Bundle By Name(cluster=T16 {"时间标识"=timestamp(0 s since 1904-01-01), "设备"="", "日志信息"="", "流程参数"=""} ("data in"), "时间标识"=w298, "设备"=w299, "日志信息"=w279, "流程参数"=w295) -> (w300:T16)
                  n176 = call "氨氮操作日志.vi"("data in"=w300) -> ()  [unwired: 11 in]
                }
              }
            }
            n177 = local write "数组"(w263) -> ()
          }
        }
      }
    }
    n178 = Not Equal?(x=w176, y=w208) -> (x != y?=w207:bool)
    n179 = call <vilib>:"Boolean Crossing PtByPt.vi"("input"=w205) -> ("crossing"=w169:bool)  [unwired: 2 in]
    n180 = Bundle By Name(cluster=T15 {"启动模式"=enum."跨度核查", "启动参数"=1, "量程"=enum."低量程"} ("参数簇"), "启动参数"=w200, "启动模式"=w202, "量程"=w201) -> (w194:T15)
    n181 = First Call?() -> (First Call?: T/F=w206:bool)
    n182 = case shown="真" w207 {
      tunnel: w176 -> [_ w418]
      frame False {
      }
      frame True {
        n183 = Subtract(x=w418, y=1) -> (x-y=w416:i32)
        n184 = Subtract(x=w416, y=5) -> (x-y=w420:i32)
        n185 = Greater Or Equal To 0?(x=w420) -> (x >= 0?=w419:bool)
        n186 = property on="多列列表框" class="MCListbox (严格)"() -> (error out=w424:errorcluster, "TopLeft"=w425:T18)  [unwired: 2 in, 1 out]
        n187 = Select(t=w420, s=w419, f=0) -> (s? t:f=w421:i32)
        n188 = Bundle By Name(cluster=w425, "Row"=w421) -> (w426:T18)
        n189 = property on="多列列表框" class="MCListbox (严格)"(error in=w424, "TopLeft"=w426) -> ()  [unwired: 1 in, 2 out]
      }
    }
    n190 = Or(x=w169, y=w206) -> (x .or. y?=w204:bool)
    n191 = while {
      tunnel: w204 -> [w404]
      tunnel: w194 -> [w403]
      shift-right: [w398] -> _
      shift-left: _ -> [w400]
      shift-right: [w399] -> _
      shift-left: _ -> [w401]
      stop <- TRUE stop-if-true
      n192 = case shown="真" w404 {
        tunnel: [w406 w414] -> w399
        tunnel: [w405 w413] -> w398
        tunnel: w403 -> [_ w408]
        tunnel: w401 -> [w406 _]
        tunnel: w400 -> [w405 _]
        frame False {
        }
        frame True {
          n193 = call "斯坦道XML解析.vi"("添加的路径"="流程路径", "参数簇"=w408) -> ("步骤时间"=w409:string[], "步骤名"=w411:string[])  [unwired: 8 in]
          n194 = for {
            tunnel: w411 -> [_] mode=indexing
            tunnel: [w415] -> w412 mode=indexing
            i -> [w415]
          }
          n195 = Build Array(w411, w409) -> (w410:string[][])
          n196 = Transpose 2D Array(2D array=w410) -> (transposed array=w413:string[][])
          n197 = Number To Decimal String(number=w412) -> (decimal integer string=w414:string[])  [unwired: 1 in]
        }
      }
      n198 = property on="多列列表框" class="MCListbox (严格)"("ItemNames"=w398, "RowHdrs[]"=w399) -> ()  [unwired: 2 in, 2 out]
    }
    n199 = case shown="1, 默认" w188 {
      selector: w188 -> [_ w345]
      tunnel: w191 -> [_ w346]
      tunnel: w190 -> [_ w344]
      frame 0 {
      }
      frame 1, Default {
        n200 = case shown="真" w344 {
          tunnel: w346 -> [_ w353]
          tunnel: w345 -> [_ w347]
          frame False {
          }
          frame True {
            n201 = case shown="默认" w347 {
              selector: w347 -> [w355 _ _ _ _ _ _ _ _ _ _ _ _ _ _ _ _ _ _ _ _ _ _ _ _ _ _ _ _ _ _ _ _ _ _ _ _ _]
              tunnel: [w354 "无告警" "缺试剂告警" "缺水样告警" "缺蒸馏水告警" "缺标液告警" "仪表漏液告警" "标定异常告警" "超量程告警" "加热异常" "低试剂预警" "超上限告警" "超下限告警" "仪表内部其他异常" "滴定异常告警" "电极异常告警" "量程切换告警" "参数设置告警" "PH电极电位异常" "电导率电极异常" "浊度光度异常" "溶解氧电极异常" "溶解氧光强异常" "温度异常告警" "PH异常告警" "溶解氧异常告警" "电导率异常告警" "浊度异常告警" "叶绿素异常告警" "藻密度异常告警" "蓝绿藻异常告警" "ORP异常告警" "氨氮异常告警" "清洁刷异常告警" "SD卡异常告警" "蓝牙异常告警" "WiFi异常告警" "流程异常告警"] -> w348
              frame Default {
                n202 = Format Into String(format string="%d" ("格式字符串"), initial string="内部告警-" ("工作状态"), w355) -> (resulting string=w354:string)  [unwired: 1 in, 1 out]
              }
              frame 0 {
              }
              frame 1 {
              }
              frame 2 {
              }
              frame 3 {
              }
              frame 4 {
              }
              frame 5 {
              }
              frame 6 {
              }
              frame 7 {
              }
              frame 8 {
              }
              frame 9 {
              }
              frame 10 {
              }
              frame 11 {
              }
              frame 12 {
              }
              frame 13 {
              }
              frame 14 {
              }
              frame 15 {
              }
              frame 16 {
              }
              frame 17 {
              }
              frame 18 {
              }
              frame 19 {
              }
              frame 20 {
              }
              frame 21 {
              }
              frame 22 {
              }
              frame 23 {
              }
              frame 24 {
              }
              frame 25 {
              }
              frame 26 {
              }
              frame 27 {
              }
              frame 28 {
              }
              frame 29 {
              }
              frame 30 {
              }
              frame 31 {
              }
              frame 32 {
              }
              frame 33 {
              }
              frame 34 {
              }
              frame 35 {
              }
              frame 36 {
              }
            }
            n203 = case shown="3, 92" w353 {
              tunnel: ["总磷" ("table输入") "氨氮" ("table输入") "总氮" ("table输入")] -> w349
              frame 1, 131 {
              }
              frame 3, 92 {
              }
              frame 2, 76, Default {
              }
            }
            n204 = Get Date/Time In Seconds() -> (seconds since 1Jan1904=w350:timestamp)
            n205 = Bundle By Name(cluster=T17 {"时间标识"=timestamp(0 s since 1904-01-01), "设备"="", "日志信息"=""} ("data in"), "时间标识"=w350, "设备"=w349, "日志信息"=w348) -> (w351:T17)
            n206 = call "氨氮报警信息.vi"("data in"=w351) -> ()  [unwired: 10 in, 1 out]
          }
        }
      }
    }
  }
  n207 = while {
    tunnel: w10 -> [w431]
    tunnel: [w429] -> _
    stop <- FALSE stop-if-true
    # "定时更新"
    n208 = Get Queue Status(queue=w431) -> (queue out=w428:refnum<queue>, # elements in queue=w427:i32)  [unwired: 2 in, 6 out]
    n209 = case shown="0" w427 {
      tunnel: [_ w434] -> w429
      tunnel: w428 -> [_ w433]
      frame Default {
      }
      frame 0 {
        w437 = u16 3 items=["总磷"=1, "氨氮"=3] ("站号")
        n210 = call "版本号读取.vi"() -> ("error out"=w434:errorcluster, "固件版本号"=→"固件版本号":string)  [unwired: 10 in]
        n211 = Bundle By Name(cluster=cluster{"命令":string, "data":variant} {"命令"="", "data"=variant} ("元素"), "命令"="读序列号", "data"=w437) -> (w436:cluster{"命令":string, "data":variant})
        n212 = Enqueue Element(queue=w433, element=w436) -> ()  [unwired: 2 in, 3 out]
      }
    }
    n213 = Wait (ms)(milliseconds to wait=u32 1000 ("等待时间（毫秒）")) -> ()  [unwired: 1 out]
  }
  n214 = property on="曲线模型" class="曲线模型 (严格)"("属性"=w1) -> (error out=w9:errorcluster)  [unwired: 2 in, 1 out]
  n215 = Cancel Notification(0:w6) -> (8:w5:refnum<notifier>)  [unwired: 1 in, 2 out]
  n216 = Obtain Queue(name (unnamed)="NH3N" ("名称（未命名）"), element data type=cluster{"命令":string, "data":variant} {"命令"="", "data"=variant}) -> (queue out=w20:refnum<queue>, error out=w21:errorcluster)  [unwired: 3 in, 1 out]
  n217 = while {
    tunnel: w20 -> [w445]
    tunnel: w21 -> [_]
    stop <- FALSE stop-if-true
    n218 = Get Queue Status(queue=w445) -> (queue out=w441:refnum<queue>, # elements in queue=w440:i32)  [unwired: 2 in, 6 out]
    n219 = Wait (ms)(milliseconds to wait=u32 1000 ("等待时间（毫秒）")) -> ()  [unwired: 1 out]
    n220 = global read "氨氮断电保存全局变量.vi" "流程路径"() -> (w444:path)
    n221 = case shown="0" w440 {
      tunnel: w441 -> [_ w448]
      frame Default {
      }
      frame 0 {
        w457 = u16 3 items=["总磷"=1, "氨氮"=3] ("站号")
        # "试剂填充 172 \n管路清洗108\n氨氮92\n总磷131\n总磷海水147\n总氮76\n总氮海水92"
        n222 = global read "VAR氨氮全局变量.vi" "状态告警区"() -> (w449:T4)
        n223 = Bundle By Name(cluster=cluster{"命令":string, "data":variant} {"命令"="", "data"=variant} ("元素"), "命令"="读状态告警区", "data"=w457) -> (w463:cluster{"命令":string, "data":variant})
        n224 = Bundle By Name(cluster=cluster{"命令":string, "data":variant} {"命令"="", "data"=variant} ("元素"), "命令"="读测量数据区", "data"=w457) -> (w460:cluster{"命令":string, "data":variant})
        n225 = Unbundle By Name(w449) -> ("系统时间"=w456:timestamp)
        n226 = Enqueue Element(queue=w448, element=w463) -> (queue out=w458:refnum<queue>)  [unwired: 2 in, 2 out]
        n227 = Get Date/Time In Seconds() -> (seconds since 1Jan1904=w455:timestamp)
        n228 = Subtract(x=w455, y=w456) -> (x-y=w454:dbl)
        n229 = Absolute Value(x=w454) -> (abs(x)=w453:dbl)
        n230 = Enqueue Element(queue=w458, element=w460) -> (queue out=w450:refnum<queue>)  [unwired: 2 in, 2 out]
        n231 = Greater Or Equal?(x=w453, y=120.0) -> (x >= y?=w451:bool)
        n232 = case shown="真" w451 {
          tunnel: w450 -> [_ w466]
          frame False {
          }
          frame True {
            n233 = call "氨氮启动命令.vi"("参数"=T19 {"站号"=3, "量程切换"=enum."AUTO", "控制命令"=enum."校时", "模式设置"=enum."待机", "测量间隔"=0}) -> ("启动命令"=w465:cluster{"命令":string, "data":variant})  [unwired: 10 in]
            n234 = Enqueue Element(queue=w466, element=w465) -> ()  [unwired: 2 in, 3 out]
          }
        }
      }
    }
    n235 = local write "流程路径"(w444) -> ()
    n236 = global read "氨氮断电保存全局变量.vi" "MB通信方式选择"() -> (w442:enum16{"串口", "TCP"})
    n237 = case shown="\"TCP\"" w442 {
      tunnel: [w468 w469] -> w443
      frame "串口", Default {
        n238 = global read "氨氮断电保存全局变量.vi" "VISA Resource"() -> (w468:refnum<visa-resource-name>)
      }
      frame "TCP" {
        n239 = global read "氨氮断电保存全局变量.vi" "IP"() -> (w469:string)
      }
    }
    "字符串" <- w443
  }
  n240 = control-ref of="测量模式下拉列表"() -> (w17:refnum<vi>)
  n241 = control-ref of="量程切换阈值"() -> (w15:refnum<vi>)
  n242 = control-ref of="参数下拉列表"() -> (w18:refnum<vi>)
  n243 = control-ref of="量程下拉列表"() -> (w19:refnum<vi>)
  n244 = control-ref of="备用系数"() -> (w14:refnum<vi>)
  n245 = control-ref of="公式"() -> (w16:refnum<vi>)
  n246 = while {
    tunnel: w20 -> [w477]
    tunnel: w19 -> [w476]
    tunnel: w18 -> [w475]
    tunnel: w17 -> [w474]
    tunnel: w16 -> [w473]
    tunnel: w15 -> [w472]
    tunnel: w14 -> [w471]
    tunnel: w9 -> [_]
    tunnel: w5 -> [w470]
    stop <- FALSE stop-if-true
    n247 = event shown="[23] \"备用系数写入\": 值改变" {
      selector: _ -> [_ _ _ _ _ _ _ _ _ _ _ _ _ _ _ _ _ _ _ _ _ _ _ _]
      dyn-events: _ -> [_ _ _ _ _ _ _ _ _ _ _ _ _ _ _ _ _ _ _ _ _ _ _ _]
      timeout: _ -> [_ _ _ _ _ _ _ _ _ _ _ _ _ _ _ _ _ _ _ _ _ _ _ _]
      tunnel: w477 -> [_ _ w493 w521 _ _ _ _ _ _ _ w624 _ w649 w656 _ _ _ _ _ _ _ _ _]
      tunnel: w476 -> [_ _ _ _ _ _ _ _ _ _ _ _ _ _ _ _ _ _ w672 _ w692 w701 w707 w719]
      tunnel: w475 -> [_ _ _ _ _ _ _ _ _ _ _ _ _ _ _ _ _ _ w670 _ w690 w703 w715 w726]
      tunnel: w474 -> [_ _ _ _ _ _ _ _ _ _ _ _ _ _ _ _ _ _ w671 _ w691 w702 w709 w721]
      tunnel: w473 -> [_ _ _ _ _ _ _ _ _ _ _ _ _ _ _ _ _ _ w666 _ _ _ _ _]
      tunnel: w472 -> [_ _ _ _ _ _ _ _ _ _ _ _ _ _ _ _ _ _ _ _ w686 _ _ _]
      tunnel: w471 -> [_ _ _ _ _ _ _ _ _ _ _ _ _ _ _ _ _ _ _ _ _ _ w713 _]
      tunnel: w470 -> [_ _ _ _ _ _ _ _ _ _ _ _ _ _ w652 _ _ _ _ _ _ _ _ _]
      tunnel: [_ w479 _ _ _ _ _ _ _ _ _ _ _ _ _ _ _ _ _ _ _ _ _ _] -> _
      event Timeout {
        n248 = event-data() -> ()  [unwired: 1 in, 3 out]
      }
      event "测量模式下拉列表", "量程下拉列表", "参数下拉列表": Value Change {
        n249 = event-data() -> ()  [unwired: 1 in, 6 out]
        n250 = local read "参数下拉列表"() -> (w480:enum16{"总磷", "总氮", "氨氮"})
        n251 = local read "测量模式下拉列表"() -> (w481:enum16{"水样测量", "零点核查", "跨度核查", "标样核查", "加标回收"})
        n252 = local read "量程下拉列表"() -> (w482:enum16{"低量程", "高量程"})
        n253 = Bundle("参数下拉列表"=w480, "测量模式下拉列表"=w481, "量程下拉列表"=w482) -> (w483:T14)  [unwired: 1 in]
        n254 = property on="曲线模型" class="曲线模型 (严格)"("属性"=w483) -> (error out=w479:errorcluster)  [unwired: 2 in, 1 out]
      }
      event "串口设置": Value Change {
        n255 = event-data() -> ()  [unwired: 1 in, 6 out]
        n256 = global read "氨氮断电保存全局变量.vi" "MB通信方式选择"() -> (w484:enum16{"串口", "TCP"})
        n257 = global read "氨氮断电保存全局变量.vi" "VISA Resource"() -> (w490:refnum<visa-resource-name>)
        n258 = global read "氨氮断电保存全局变量.vi" "PORT"() -> (w488:string)
        n259 = global read "氨氮断电保存全局变量.vi" "IP"() -> (w489:string)
        n260 = call "串口配置.vi"("PORT"=w488, "IP"=w489, "MB通信方式选择"=w484, "请选择串口:"=w490) -> ("PORT 2"=w486:string, "IP 2"=w487:string, "确认 2"=w491:bool, "VISA资源名称 2"=w492:refnum<visa-resource-name>, "MB通信方式选择 2"=w485:enum16{"串口", "TCP"})  [unwired: 3 in]
        n261 = case shown="真" w491 {
          tunnel: w492 -> [_ w498]
          tunnel: w493 -> [_ w497]
          tunnel: w487 -> [_ w496]
          tunnel: w486 -> [_ w495]
          tunnel: w485 -> [_ w494]
          frame False {
          }
          frame True {
            n262 = flat-sequence {
              tunnel: w498 -> [w503]
              tunnel: w497 -> [w504]
              tunnel: w496 -> [w502]
              tunnel: w495 -> [w501]
              tunnel: w494 -> [w500]
              frame #0 {
                n263 = global write "氨氮断电保存全局变量.vi" "IP"(w502) -> ()
                n264 = global write "氨氮断电保存全局变量.vi" "PORT"(w501) -> ()
                n265 = global write "氨氮断电保存全局变量.vi" "VISA Resource"(w503) -> ()
                n266 = global write "氨氮断电保存全局变量.vi" "MB通信方式选择"(w500) -> ()
                n267 = Flush Queue(queue=w504) -> (queue out=w499:refnum<queue>)  [unwired: 1 in, 2 out]
                n268 = Enqueue Element(queue=w499, element=cluster{"命令":string, "data":variant} {"命令"="启用模块", "data"=variant} ("元素")) -> ()  [unwired: 2 in, 3 out]
              }
              frame #1 {
                n269 = call <vilib>:"Application Directory.vi"() -> ("Application Directory"=w519:path)
                n270 = Build Path(base path=w519, name or relative path="data\\sys.ini" ("名称或相对路径")) -> (appended path=w517:path)
                n271 = call <vilib>:"Open Config Data.vi"("configuration file path"=w517) -> ("error out"=w513:errorcluster, "refnum"=w516:T13)  [unwired: 8 in, 1 out]
                n272 = vi-ref "氨氮断电保存全局变量.vi"() -> (w515:refnum<vi>)
                n273 = call <userlib>:"Write Panel to INI__ogtk.vi"("error in (no error)"=w513, "VI ref"=w515, "refnum"=w516) -> ("error out"=w512:errorcluster, "refnum out"=w514:T13)  [unwired: 7 in]
                n274 = call <vilib>:"Close Config Data.vi"("error in (no error)"=w512, "refnum"=w514) -> ("error out"=w507:errorcluster, "file path"=w506:path)  [unwired: 8 in]
                n275 = Open/Create/Replace File(file path (use dialog)=w506, error in=w507) -> (refnum out=w510:refnum<file>, error out=w511:errorcluster)  [unwired: 4 in, 1 out]
                n276 = Flush File(refnum=w510, error in=w511) -> (refnum out=w509:refnum<file>, error out=w508:errorcluster)
                n277 = Close File(refnum=w509, error in=w508) -> ()  [unwired: 2 out]
              }
            }
          }
        }
      }
      event "模块启用": Value Change {
        n278 = event-data() -> ("OldVal"=w522:bool)  [unwired: 1 in, 5 out]
        n279 = Flush Queue(queue=w521) -> (queue out=w520:refnum<queue>)  [unwired: 1 in, 2 out]
        n280 = case shown="假" w522 {
          tunnel: w520 -> [w523 w525]
          frame False {
            n281 = Enqueue Element(queue=w523, element=cluster{"命令":string, "data":variant} {"命令"="停用模块", "data"=variant} ("元素")) -> ()  [unwired: 2 in, 3 out]
          }
          frame True {
            n282 = Enqueue Element(queue=w525, element=cluster{"命令":string, "data":variant} {"命令"="启用模块", "data"=variant} ("元素")) -> ()  [unwired: 2 in, 3 out]
          }
        }
      }
      event "流程路径": Value Change {
        n283 = event-data() -> ()  [unwired: 1 in, 6 out]
        n284 = flat-sequence {
          frame #0 {
            n285 = local read "流程路径"() -> (w527:path)
            n286 = global write "氨氮断电保存全局变量.vi" "流程路径"(w527) -> ()
          }
          frame #1 {
            n287 = call <vilib>:"Application Directory.vi"() -> ("Application Directory"=w541:path)
            n288 = Build Path(base path=w541, name or relative path="data\\sys.ini" ("名称或相对路径")) -> (appended path=w539:path)
            n289 = call <vilib>:"Open Config Data.vi"("configuration file path"=w539) -> ("error out"=w535:errorcluster, "refnum"=w538:T13)  [unwired: 8 in, 1 out]
            n290 = vi-ref "氨氮断电保存全局变量.vi"() -> (w537:refnum<vi>)
            n291 = call <userlib>:"Write Panel to INI__ogtk.vi"("error in (no error)"=w535, "VI ref"=w537, "refnum"=w538) -> ("error out"=w534:errorcluster, "refnum out"=w536:T13)  [unwired: 7 in]
            n292 = call <vilib>:"Close Config Data.vi"("error in (no error)"=w534, "refnum"=w536) -> ("error out"=w529:errorcluster, "file path"=w528:path)  [unwired: 8 in]
            n293 = Open/Create/Replace File(file path (use dialog)=w528, error in=w529) -> (refnum out=w532:refnum<file>, error out=w533:errorcluster)  [unwired: 4 in, 1 out]
            n294 = Flush File(refnum=w532, error in=w533) -> (refnum out=w531:refnum<file>, error out=w530:errorcluster)
            n295 = Close File(refnum=w531, error in=w530) -> ()  [unwired: 2 out]
          }
        }
      }
      event "公式一键写入": Value Change {
        n296 = event-data() -> ()  [unwired: 1 in, 6 out]
        n297 = local read "公式"() -> (w542:cluster{"X^2":dbl, "X":dbl, "b":dbl})
        n298 = call "公式复合写入.vi"("公式"=w542) -> ()  [unwired: 11 in]
      }
      event "备用系数一键写入": Value Change {
        n299 = event-data() -> ()  [unwired: 1 in, 6 out]
        n300 = local read "备用系数"() -> (w543:T2)
        n301 = call "量程参数复合参数写入.vi"("备用系数"=w543) -> ()  [unwired: 11 in]
      }
      event "曲线模型": Value Change {
        n302 = event-data() -> ()  [unwired: 1 in, 6 out]
        n303 = local write "公式"("曲线模型") -> ()
      }
      event "质控参数设置": Value Change {
        n304 = event-data() -> ()  [unwired: 1 in, 6 out]
        n305 = global read "氨氮断电保存全局变量.vi" "质控参数设置"() -> (w545:T20)
        n306 = call "氨氮质控参数设置.vi"("质控参数设置"=w545) -> ("输出簇"=w546:T21)  [unwired: 10 in]
        n307 = Unbundle By Name(w546) -> ("确定"=w547:bool)
        n308 = case shown="真" w547 {
          tunnel: w546 -> [_ w549]
          tunnel: w545 -> [_ w548]
          frame False {
          }
          frame True {
            n309 = flat-sequence {
              tunnel: w549 -> [w556]
              tunnel: w548 -> [w555]
              frame #0 {
                n310 = Unbundle By Name(w556) -> ("跨度值"=w554:dbl, "零点标准液浓度"=w553:dbl, "跨度标准液浓度"=w552:dbl, "标准液标准浓度"=w551:dbl)
                n311 = Bundle By Name(cluster=w555, "氨氮跨度值"=w554, "氨氮零点标准液浓度"=w553, "氨氮跨度标准液浓度"=w552, "氨氮标准液标准浓度"=w551) -> (w550:T20)
                n312 = global write "氨氮断电保存全局变量.vi" "质控参数设置"(w550) -> ()
              }
              frame #1 {
                n313 = call <vilib>:"Application Directory.vi"() -> ("Application Directory"=w570:path)
                n314 = Build Path(base path=w570, name or relative path="data\\sys.ini" ("名称或相对路径")) -> (appended path=w568:path)
                n315 = call <vilib>:"Open Config Data.vi"("configuration file path"=w568) -> ("error out"=w564:errorcluster, "refnum"=w567:T13)  [unwired: 8 in, 1 out]
                n316 = vi-ref "氨氮断电保存全局变量.vi"() -> (w566:refnum<vi>)
                n317 = call <userlib>:"Write Panel to INI__ogtk.vi"("error in (no error)"=w564, "VI ref"=w566, "refnum"=w567) -> ("error out"=w563:errorcluster, "refnum out"=w565:T13)  [unwired: 7 in]
                n318 = call <vilib>:"Close Config Data.vi"("error in (no error)"=w563, "refnum"=w565) -> ("error out"=w558:errorcluster, "file path"=w557:path)  [unwired: 8 in]
                n319 = Open/Create/Replace File(file path (use dialog)=w557, error in=w558) -> (refnum out=w561:refnum<file>, error out=w562:errorcluster)  [unwired: 4 in, 1 out]
                n320 = Flush File(refnum=w561, error in=w562) -> (refnum out=w560:refnum<file>, error out=w559:errorcluster)
                n321 = Close File(refnum=w560, error in=w559) -> ()  [unwired: 2 out]
              }
            }
          }
        }
      }
      event "仪器参数设置": Value Change {
        n322 = event-data() -> ()  [unwired: 1 in, 6 out]
        n323 = global read "氨氮断电保存全局变量.vi" "氨氮仪器参数"() -> (w572:T22)
        n324 = call "仪器参数设置.vi"("仪器参数设置"=w572) -> ("仪器参数设置输出"=w571:T23)  [unwired: 10 in]
        n325 = Unbundle By Name(w571) -> ("确定"=w573:bool)
        n326 = case shown="真" w573 {
          tunnel: w571 -> [_ w575]
          tunnel: w572 -> [_ w574]
          frame False {
          }
          frame True {
            n327 = flat-sequence {
              tunnel: w575 -> [w592]
              tunnel: w574 -> [w591]
              frame #0 {
                n328 = Unbundle By Name(w592) -> ("测量量程"=w590:dbl, "测量精度"=w589:dbl, "测量间隔"=w588:dbl, "消解温度"=w587:dbl, "消解时长"=w585:dbl, "空白校准时间"=w584:timestamp, "曲线截距"=w583:dbl, "曲线斜率"=w582:dbl, "测量检出限"=w581:dbl, "测量信号值"=w580:dbl, "线性相关系数"=w579:dbl, "二次多项式系数"=w578:dbl, "标样校准时间"=w577:timestamp, "单位"=w576:u16)
                n329 = Bundle By Name(cluster=w591, "测量量程"=w590, "测量精度"=w589, "测量间隔"=w588, "消解温度"=w587, "消解时长"=w585, "空白校准时间"=w584, "曲线截距"=w583, "曲线斜率"=w582, "测量检出限"=w581, "测量信号值"=w580, "线性相关系数"=w579, "二次多项式系数"=w578, "标样校准时间"=w577, "单位"=w576) -> (w586:T22)
                n330 = global write "氨氮断电保存全局变量.vi" "氨氮仪器参数"(w586) -> ()
              }
              frame #1 {
                n331 = call <vilib>:"Application Directory.vi"() -> ("Application Directory"=w606:path)
                n332 = Build Path(base path=w606, name or relative path="data\\sys.ini" ("名称或相对路径")) -> (appended path=w604:path)
                n333 = call <vilib>:"Open Config Data.vi"("configuration file path"=w604) -> ("error out"=w600:errorcluster, "refnum"=w603:T13)  [unwired: 8 in, 1 out]
                n334 = vi-ref "氨氮断电保存全局变量.vi"() -> (w602:refnum<vi>)
                n335 = call <userlib>:"Write Panel to INI__ogtk.vi"("error in (no error)"=w600, "VI ref"=w602, "refnum"=w603) -> ("error out"=w599:errorcluster, "refnum out"=w601:T13)  [unwired: 7 in]
                n336 = call <vilib>:"Close Config Data.vi"("error in (no error)"=w599, "refnum"=w601) -> ("error out"=w594:errorcluster, "file path"=w593:path)  [unwired: 8 in]
                n337 = Open/Create/Replace File(file path (use dialog)=w593, error in=w594) -> (refnum out=w597:refnum<file>, error out=w598:errorcluster)  [unwired: 4 in, 1 out]
                n338 = Flush File(refnum=w597, error in=w598) -> (refnum out=w596:refnum<file>, error out=w595:errorcluster)
                n339 = Close File(refnum=w596, error in=w595) -> ()  [unwired: 2 out]
              }
            }
          }
        }
      }
      event "自动测试量程配置": Value Change {
        n340 = event-data() -> ()  [unwired: 1 in, 6 out]
        n341 = flat-sequence {
          frame #0 {
            n342 = global write "氨氮断电保存全局变量.vi" "氨氮自动测试量程配置"("自动测试量程配置") -> ()
          }
          frame #1 {
            n343 = call <vilib>:"Application Directory.vi"() -> ("Application Directory"=w621:path)
            n344 = Build Path(base path=w621, name or relative path="data\\sys.ini" ("名称或相对路径")) -> (appended path=w619:path)
            n345 = call <vilib>:"Open Config Data.vi"("configuration file path"=w619) -> ("error out"=w615:errorcluster, "refnum"=w618:T13)  [unwired: 8 in, 1 out]
            n346 = vi-ref "氨氮断电保存全局变量.vi"() -> (w617:refnum<vi>)
            n347 = call <userlib>:"Write Panel to INI__ogtk.vi"("error in (no error)"=w615, "VI ref"=w617, "refnum"=w618) -> ("error out"=w614:errorcluster, "refnum out"=w616:T13)  [unwired: 7 in]
            n348 = call <vilib>:"Close Config Data.vi"("error in (no error)"=w614, "refnum"=w616) -> ("error out"=w609:errorcluster, "file path"=w608:path)  [unwired: 8 in]
            n349 = Open/Create/Replace File(file path (use dialog)=w608, error in=w609) -> (refnum out=w612:refnum<file>, error out=w613:errorcluster)  [unwired: 4 in, 1 out]
            n350 = Flush File(refnum=w612, error in=w613) -> (refnum out=w611:refnum<file>, error out=w610:errorcluster)
            n351 = Close File(refnum=w611, error in=w610) -> ()  [unwired: 2 out]
          }
        }
      }
      event "手动启动": Value Change {
        n352 = event-data() -> ()  [unwired: 1 in, 6 out]
        n353 = call "氨氮启动参数对话框.vi"() -> ("确认"=w622:bool, "元素"=w623:cluster{"命令":string, "data":variant})  [unwired: 10 in]
        n354 = case shown="真" w622 {
          tunnel: w624 -> [_ w626]
          tunnel: w623 -> [_ w625]
          frame False {
          }
          frame True {
            n355 = Enqueue Element(queue=w626, element=w625) -> ()  [unwired: 2 in, 3 out]
          }
        }
      }
      event "定时启动": Mouse Down {
        n356 = event-data() -> ()  [unwired: 1 in, 6 out]
        n357 = flat-sequence {
          frame #0 {
            n358 = global read "氨氮断电保存全局变量.vi" "定时控制"() -> (w628:T6)
            n359 = call "周期设置.vi"("定时控制输入"=w628) -> ("定时控制输出"=w627:T24)  [unwired: 10 in]
            n360 = global write "氨氮断电保存全局变量.vi" "定时控制"(w627) -> ()
          }
          frame #1 {
            n361 = call <vilib>:"Application Directory.vi"() -> ("Application Directory"=w642:path)
            n362 = Build Path(base path=w642, name or relative path="data\\sys.ini" ("名称或相对路径")) -> (appended path=w640:path)
            n363 = call <vilib>:"Open Config Data.vi"("configuration file path"=w640) -> ("error out"=w636:errorcluster, "refnum"=w639:T13)  [unwired: 8 in, 1 out]
            n364 = vi-ref "氨氮断电保存全局变量.vi"() -> (w638:refnum<vi>)
            n365 = call <userlib>:"Write Panel to INI__ogtk.vi"("error in (no error)"=w636, "VI ref"=w638, "refnum"=w639) -> ("error out"=w635:errorcluster, "refnum out"=w637:T13)  [unwired: 7 in]
            n366 = call <vilib>:"Close Config Data.vi"("error in (no error)"=w635, "refnum"=w637) -> ("error out"=w630:errorcluster, "file path"=w629:path)  [unwired: 8 in]
            n367 = Open/Create/Replace File(file path (use dialog)=w629, error in=w630) -> (refnum out=w633:refnum<file>, error out=w634:errorcluster)  [unwired: 4 in, 1 out]
            n368 = Flush File(refnum=w633, error in=w634) -> (refnum out=w632:refnum<file>, error out=w631:errorcluster)
            n369 = Close File(refnum=w632, error in=w631) -> ()  [unwired: 2 out]
          }
        }
      }
      event "单步测试": Value Change {
        w644 = u16 1 items=["总磷"=1, "氨氮"=3] ("站号")
        n370 = event-data() -> ()  [unwired: 1 in, 6 out]
        n371 = Bundle("站号"=w644, "总磷氨氮调试"="总磷氨氮调试") -> (w643:cluster{"站号":u16, "总磷氨氮调试":u16[]})  [unwired: 1 in]
        n372 = Bundle By Name(cluster=cluster{"命令":string, "data":variant} {"命令"="", "data"=variant} ("元素"), "命令"="debug", "data"=w643) -> (w646:cluster{"命令":string, "data":variant})
        n373 = Enqueue Element(queue=w649, element=w646) -> ()  [unwired: 2 in, 3 out]
      }
      event "停止": Value Change {
        n374 = event-data() -> ()  [unwired: 1 in, 6 out]
        n375 = Enqueue Element(queue=w656, element=cluster{"命令":string, "data":variant} {"命令"="启动", "data"=variant(cluster{"站号":u16, "控制命令输出":u16[]} {"站号"=1, "控制命令输出"=[2816]})} ("元素")) -> (queue out=w654:refnum<queue>)  [unwired: 2 in, 2 out]
        n376 = Cancel Notification(0:w652) -> (8:w653:refnum<notifier>)  [unwired: 1 in, 2 out]
        n377 = Send Notification(notification=TRUE ("通知"), notifier=w653) -> ()  [unwired: 1 in, 2 out]
        n378 = Enqueue Element(queue=w654, element=cluster{"命令":string, "data":variant} {"命令"="启动", "data"=variant(cluster{"站号":u16, "控制命令":u16[]} {"站号"=3, "控制命令"=[2816]})} ("启动命令")) -> ()  [unwired: 2 in, 3 out]
      }
      event "设置": Value Change {
        n379 = event-data() -> ()  [unwired: 1 in, 6 out]
        n380 = property on="窗格" class="Pane"("Origin"=T11 {"Horizontal"=0, "Vertical"=628} ("原点")) -> ()  [unwired: 2 in, 2 out]
      }
      event "返回": Value Change {
        n381 = event-data() -> ()  [unwired: 1 in, 6 out]
        n382 = property on="窗格" class="Pane"("Origin"=T11 {"Horizontal"=0, "Vertical"=0} ("原点")) -> ()  [unwired: 2 in, 2 out]
      }
      event "公式.X^2", "公式.X", "公式.b", "量程切换阈值.阈值", "量程切换阈值.标液浓度", "备用系数.量程上限", "备用系数.量程下限", "备用系数.检出限", "备用系数.精度": Mouse Down {
        n383 = event-data() -> ("CtlRef"=w662:refnum<vi>)  [unwired: 1 in, 5 out]
        n384 = property class="DigNum (严格)"(reference=w662) -> (reference out=w660:refnum<vi>, "Value"=w661:dbl)  [unwired: 1 in, 1 out]
        n385 = call "数字键盘.vi"("OldNumber"=w661) -> ("NewNumber"=w659:dbl)
        n386 = property class="DigNum (严格)"(reference=w660, "Val(Sgnl)"=w659) -> ()  [unwired: 1 in, 2 out]
      }
      event "读公式": Value Change {
        n387 = event-data() -> ()  [unwired: 1 in, 6 out]
        n388 = property class="Enum (严格)"(reference=w670) -> ("Value"=w669:enum16{"总磷", "总氮", "氨氮"})  [unwired: 1 in, 2 out]
        n389 = property class="Enum (严格)"(reference=w671) -> ("Value"=w668:enum16{"水样测量", "零点核查", "跨度核查", "标样核查", "加标回收"})  [unwired: 1 in, 2 out]
        n390 = property class="Enum (严格)"(reference=w672) -> ("Value"=w667:enum16{"低量程", "高量程"})  [unwired: 1 in, 2 out]
        n391 = call "公式读取.vi"("量程"=w667, "测量模式"=w668, "测量参数"=w669) -> ("error out"=w664:errorcluster, "公式"=w665:cluster{"X^2":dbl, "X":dbl, "b":dbl})  [unwired: 7 in]
        n392 = property class="Clust (严格)"(reference=w666, "Value"=w665) -> ()  [unwired: 1 in, 2 out]
        n393 = case shown="错误" w664 {
          tunnel: ["读取成功" ("消息") "读取失败" ("消息")] -> w663
          frame No Error {
          }
          frame Error {
          }
        }
        n394 = One Button Dialog(message=w663) -> ()  [unwired: 1 in, 1 out]
      }
      event "写公式": Value Change {
        n395 = event-data() -> ()  [unwired: 1 in, 6 out]
        n396 = call "公式写入.vi"("公式"="公式", "量程"="量程下拉列表", "测量模式"="测量模式下拉列表", "测量参数"="参数下拉列表") -> ("error out"=w677:errorcluster)  [unwired: 7 in]
        n397 = case shown="无错误" w677 {
          tunnel: ["写入成功" ("消息") "写入失败" ("消息")] -> w678
          frame No Error {
          }
          frame Error {
          }
        }
        n398 = One Button Dialog(message=w678) -> ()  [unwired: 1 in, 1 out]
      }
      event "量程切换阈值读取": Value Change {
        n399 = event-data() -> ()  [unwired: 1 in, 6 out]
        n400 = property class="Enum (严格)"(reference=w690) -> ("Value"=w689:enum16{"总磷", "总氮", "氨氮"})  [unwired: 1 in, 2 out]
        n401 = property class="Enum (严格)"(reference=w691) -> ("Value"=w688:enum16{"水样测量", "零点核查", "跨度核查", "标样核查", "加标回收"})  [unwired: 1 in, 2 out]
        n402 = property class="Enum (严格)"(reference=w692) -> ("Value"=w687:enum16{"低量程", "高量程"})  [unwired: 1 in, 2 out]
        n403 = call "量程读取.vi"("量程"=w687, "测量模式"=w688, "测量参数"=w689) -> ("error out"=w683:errorcluster, "量程切换阈值"=w685:cluster{"阈值":dbl, "标液浓度":dbl})  [unwired: 7 in]
        n404 = property class="Clust (严格)"(reference=w686, "Value"=w685) -> ()  [unwired: 1 in, 2 out]
        n405 = case shown="错误" w683 {
          tunnel: ["读取成功" ("消息") "读取失败" ("消息")] -> w684
          frame No Error {
          }
          frame Error {
          }
        }
        n406 = One Button Dialog(message=w684) -> ()  [unwired: 1 in, 1 out]
      }
      event "量程切换阈值写入": Value Change {
        n407 = event-data() -> ()  [unwired: 1 in, 6 out]
        n408 = property class="Enum (严格)"(reference=w703) -> ("Value"=w700:enum16{"总磷", "总氮", "氨氮"})  [unwired: 1 in, 2 out]
        n409 = property class="Enum (严格)"(reference=w702) -> ("Value"=w699:enum16{"水样测量", "零点核查", "跨度核查", "标样核查", "加标回收"})  [unwired: 1 in, 2 out]
        n410 = property class="Enum (严格)"(reference=w701) -> ("Value"=w698:enum16{"低量程", "高量程"})  [unwired: 1 in, 2 out]
        n411 = call "量程写入.vi"("量程切换阈值"="量程切换阈值", "量程"=w698, "测量模式"=w699, "测量参数"=w700) -> ("error out"=w695:errorcluster)  [unwired: 7 in]
        n412 = case shown="无错误" w695 {
          tunnel: ["写入成功" ("消息") "写入失败" ("消息")] -> w696
          frame No Error {
          }
          frame Error {
          }
        }
        n413 = One Button Dialog(message=w696) -> ()  [unwired: 1 in, 1 out]
      }
      event "备用系数读取": Value Change {
        n414 = event-data() -> ()  [unwired: 1 in, 6 out]
        n415 = property class="Enum (严格)"(reference=w715) -> ("Value"=w714:enum16{"总磷", "总氮", "氨氮"})  [unwired: 1 in, 2 out]
        n416 = property class="Enum (严格)"(reference=w709) -> ("Value"=w708:enum16{"水样测量", "零点核查", "跨度核查", "标样核查", "加标回收"})  [unwired: 1 in, 2 out]
        n417 = property class="Enum (严格)"(reference=w707) -> ("Value"=w706:enum16{"低量程", "高量程"})  [unwired: 1 in, 2 out]
        n418 = call "备用系数读取.vi"("量程"=w706, "测量模式"=w708, "测量参数"=w714) -> ("error out"=w710:errorcluster, "备用系数"=w712:T2)  [unwired: 7 in]
        n419 = property class="Clust (严格)"(reference=w713, "Value"=w712) -> ()  [unwired: 1 in, 2 out]
        n420 = case shown="错误" w710 {
          tunnel: ["读取成功" ("消息") "读取失败" ("消息")] -> w711
          frame No Error {
          }
          frame Error {
          }
        }
        n421 = One Button Dialog(message=w711) -> ()  [unwired: 1 in, 1 out]
      }
      event "备用系数写入": Value Change {
        n422 = event-data() -> ()  [unwired: 1 in, 6 out]
        n423 = property class="Enum (严格)"(reference=w726) -> ("Value"=w725:enum16{"总磷", "总氮", "氨氮"})  [unwired: 1 in, 2 out]
        n424 = property class="Enum (严格)"(reference=w721) -> ("Value"=w720:enum16{"水样测量", "零点核查", "跨度核查", "标样核查", "加标回收"})  [unwired: 1 in, 2 out]
        n425 = property class="Enum (严格)"(reference=w719) -> ("Value"=w718:enum16{"低量程", "高量程"})  [unwired: 1 in, 2 out]
        n426 = call "备用系数写入.vi"("备用系数"="备用系数", "量程"=w718, "测量模式"=w720, "测量参数"=w725) -> ("error out"=w722:errorcluster)  [unwired: 7 in]
        n427 = case shown="无错误" w722 {
          tunnel: ["写入成功" ("消息") "写入失败" ("消息")] -> w723
          frame No Error {
          }
          frame Error {
          }
        }
        n428 = One Button Dialog(message=w723) -> ()  [unwired: 1 in, 1 out]
      }
    }
  }
